vi "VISA read.vi"(8 "error in (no error)":errorcluster, 11 "Cobolt in":refnum<class "Cobolt.lvclass">) -> (0 "error out":errorcluster, 2 "buffer out":string, 3 "Cobolt out":refnum<class "Cobolt.lvclass">)   [LabVIEW 2012, in "Cobolt.lvclass"]
uses:
  Cobolt.lvclass
  Cobolt.lvclass/Cobolt.ctl
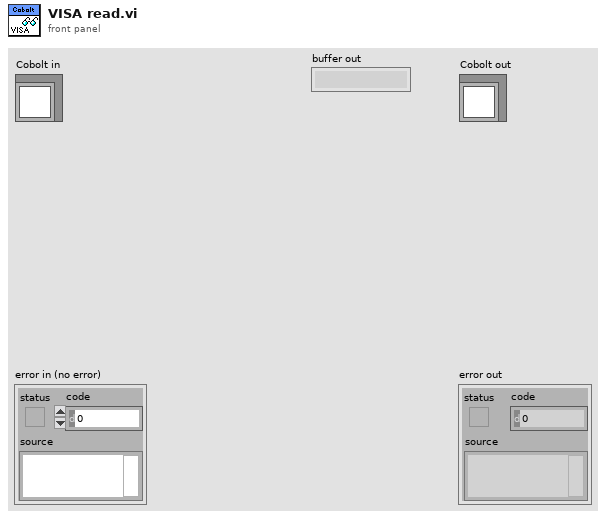
[diagram p1: front panel]
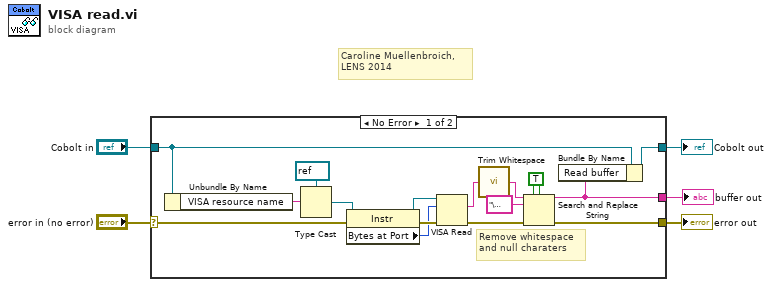
[diagram p0: block diagram]
diagram:
  # "Caroline Muellenbroich, \nLENS 2014"
  n1 = case shown="No Error" "error in (no error)" {
    selector: "error in (no error)" -> [w13 w23]
    tunnel: [w8 w23] -> w4
    tunnel: [w14 w22] -> w2
    tunnel: "Cobolt in" -> [w15 w22]
    tunnel: [w7 _] -> w1
    frame No Error {
      w12 = TRUE ("replace all? (F)")
      # "Remove whitespace\nand null charaters"
      n2 = Unbundle By Name(w15) -> ("VISA resource name"=w17:string)
      n3 = Type Cast(type=refnum<visa-resource-name> refnum ("reference"), x=w17) -> (*(type *) &x=w16:refnum<visa-resource-name>)
      n4 = property class="Instr"(reference=w16, error in=w13) -> (reference out=w20:refnum<visa-resource-name>, error out=w21:errorcluster, "Bytes at Port"=w19:u32)
      n5 = VISA Read(VISA resource name=w20, byte count=w19, error in (no error)=w21) -> (read buffer=w6:string, error out=w9:errorcluster)  [unwired: 2 out]
      n6 = call <vilib>:"Trim Whitespace.vi"("string"=w6) -> ("trimmed string"=w10:string)  [unwired: 1 in]
      n7 = Search and Replace String(replace all?=w12, case sensitive?=w12, input string=w10, search string="\u0000", error in=w9) -> (result string=w7:string, error out=w8:errorcluster)  [unwired: 3 in, 2 out]
      n8 = Bundle By Name(cluster=w15, "Read buffer"=w7) -> (w14:refnum<class "Cobolt.lvclass">)
    }
    frame Error {
    }
  }
  "error out" <- w4
  "Cobolt out" <- w2
  "buffer out" <- w1
